vi "PN to poly scripter.vi"   [LabVIEW 2015]
uses:
  SLSC Interface.lvclass
types:
  T1 = enum32{"invalid VI type", "Standard VI", "Control VI", "Global VI", "Polymorphic VI", "Configuration VI", "SubSystem", "Facade VI", "Method VI", "Statechart Diagram VI"}
  T2 = cluster{"appended path":path, "Short name (localized)":string, "Long name (localized)":string}[]
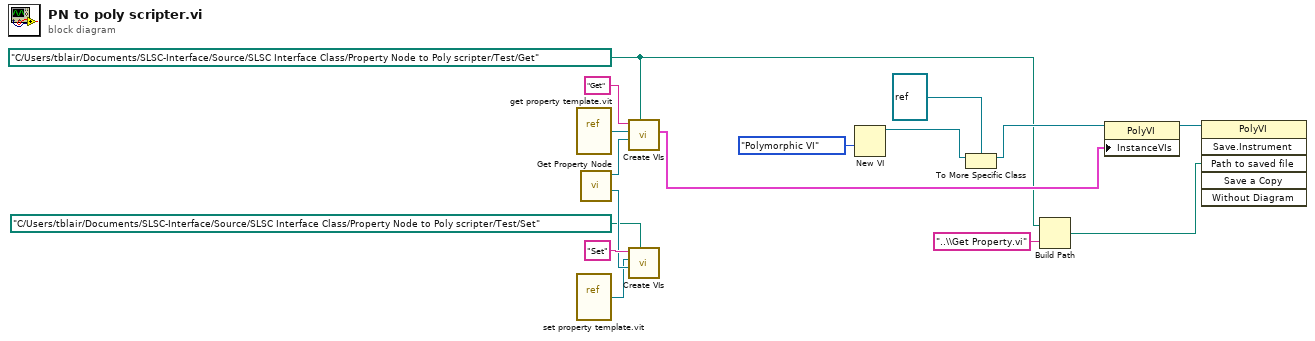
[diagram p0: block diagram]
diagram:
  w3 = path "C:/Users/tblair/Documents/SLSC-Interface/Source/SLSC Interface Class/Property Node to Poly scripter/Test/Get" ("Path")
  n1 = vi-ref "get property template.vit"() -> (w16:refnum<vi>)
  n2 = vi-ref "set property template.vit"() -> (w11:refnum<vi>)
  n3 = call "Get Property Node.vi"() -> ("Write Property out"=w12:refnum<vi>, "Read Property out"=w15:refnum<vi>)  [unwired: 9 in, 1 out]
  n4 = call "Create VIs.vi"("Path"=w3, "Property in"=w15, "Template"=w16, "prefix"="Get") -> ("Poly Info"=w5:T2)  [unwired: 7 in]
  n5 = call "Create VIs.vi"("Path"=path "C:/Users/tblair/Documents/SLSC-Interface/Source/SLSC Interface Class/Property Node to Poly scripter/Test/Set", "Property in"=w12, "Template"=w11, "prefix"="Set") -> ()  [unwired: 7 in, 1 out]
  n6 = New VI(9:T1."Polymorphic VI" ("vi type (standard vi)")) -> (3:w8:refnum<vi>)  [unwired: 6 in, 1 out]
  n7 = To More Specific Class(target class=refnum<vi> refnum, reference=w8) -> (specific class reference=w6:refnum<vi>)  [unwired: 1 in, 1 out]
  n8 = Build Path(base path=w3, name or relative path="..\\Get Property.vi") -> (appended path=w1:path)
  n9 = property class="PolyVI"(reference=w6, "InstanceVIs"=w5) -> (reference out=w4:refnum<vi>)  [unwired: 1 in, 1 out]
  n10 = invoke class="PolyVI" method="Save.Instrument"(reference=w4, "Path to saved file"=w1) -> ()  [unwired: 4 in, 6 out]
